vi "Get Scaled BD to Pic File.vi"(6 "选择文件类型":enum16{"PNG", "JPG", "BMP"}(ring), 8 "错误输入（无错误）":errorcluster, 9 "图片文件存储路径":path, 10 "图像参数":cluster{"图像深度":i32, "最大宽度":i32, "最大高度":i32}={"图像深度"=8, "最大宽度"=0, "最大高度"=0} {"图像深度" items=["1位、黑白"=1, "4位、16色"=4, "8位、256色"=8, "24位、真彩色"=24]}, 11 "VI Ref":refnum<vi>) -> (0 "错误输出":errorcluster)   [LabVIEW 2012, in "VIRef.lvlib"]
uses:
  VIRef.lvlib
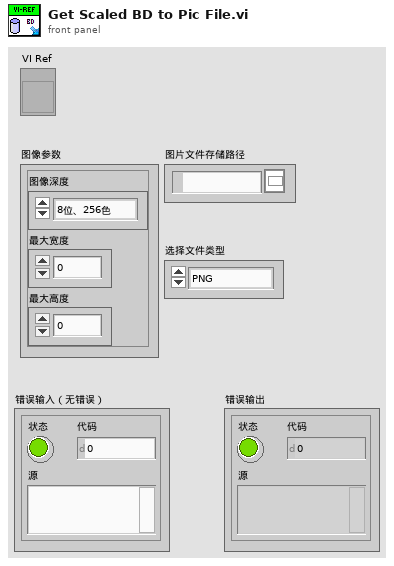
[diagram p1: front panel]
types:
  T1 = typedef "imagedata.ctl" = cluster{"image type":i32, "image depth":i32, "image":u8[], "mask":u8[], "colors":u32[], "Rectangle":cluster{"left":i16, "top":i16, "right":i16, "bottom":i16}}
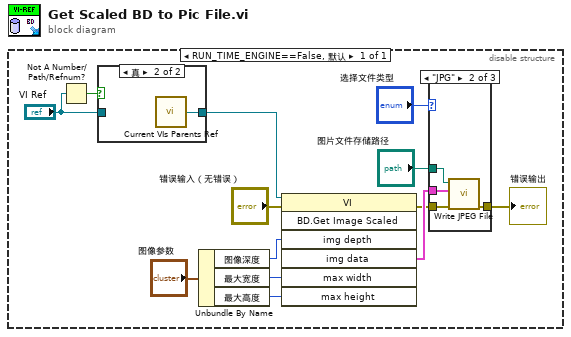
[diagram p0: block diagram]
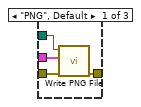
[diagram p2: hidden frame]
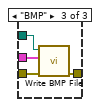
[diagram p3: hidden frame]
diagram:
  n1 = disable-structure shown="RUN_TIME_ENGINE==False, 默认" {
    frame condition #0 (active) {
      n2 = Not A Number/Path/Refnum?(number/path/refnum="VI Ref") -> (NaN/Path/Refnum?=w13:bool)
      n3 = case shown="真" w13 {
        tunnel: [w26 w27] -> w11
        tunnel: "VI Ref" -> [w26 _]
        frame False {
        }
        frame True {
          n4 = call "Current VIs Parents Ref.vi"() -> ("Calling VI's Reference"=w27:refnum<vi>)  [unwired: 2 in]
        }
      }
      n5 = Unbundle By Name("图像参数") -> ("图像深度"=w8:i32, "最大宽度"=w7:i32, "最大高度"=w6:i32)
      n6 = invoke class="VI" method="BD.Get Image Scaled"(reference=w11, error in="错误输入（无错误）", "img depth"=w8, "max width"=w7, "max height"=w6) -> (error out=w2:errorcluster, "img data"=w3:T1)  [unwired: 2 in, 5 out]
      n7 = case shown="\"JPG\"" "选择文件类型" {
        tunnel: "图片文件存储路径" -> [w14 w18 w23]
        tunnel: w3 -> [w15 w21 w22]
        tunnel: w2 -> [w17 w20 w25]
        tunnel: [w16 w19 w24] -> w1
        frame "PNG", Default {
          n8 = call <vilib>:"Write PNG File.vi"("error in (no error)"=w17, "image data"=w15, "path to PNG file"=w14) -> ("error out"=w16:errorcluster)  [unwired: 7 in, 1 out]
        }
        frame "JPG" {
          n9 = call <vilib>:"Write JPEG File.vi"("error in (no error)"=w20, "image data"=w21, "path to JPEG file"=w18) -> ("error out"=w19:errorcluster)  [unwired: 7 in, 1 out]
        }
        frame "BMP" {
          n10 = call <vilib>:"Write BMP File.vi"("error in (no error)"=w25, "image data"=w22, "path to BMP file"=w23) -> ("error out"=w24:errorcluster)  [unwired: 7 in, 1 out]
        }
      }
      "错误输出" <- w1
    }
  }
